vi "WaveSynthV2.vi"(6 "error in":errorcluster, 9 "Default Wave":bool) -> (0 "error out":errorcluster, 1 "Waves per Pixel 2":u32, 2 "Sampling Frequency (Hz) 2":u64, 3 "Amplitudes":dbl[](array[numeric]) format="%.2f", 4 "Offset Factor 2":dbl, 5 "Gain":dbl)   [LabVIEW 2020]
uses:
  WaveFormsAvailable.ctl
  <vilib>/Utility/file.llb/Read Delimited Spreadsheet (DBL).vi
  <vilib>/Utility/file.llb/Write Delimited Spreadsheet (DBL).vi
  <vilib>/Analysis/NI_AALBase.lvlib
panel:
  in  "Developers Option Control":enum32{"Dev"}(tab)
  out "Time Series":dbl[](array[numeric])
  in  "Wave View":enum32{"Single", "Complete Wave"}(tab)
  out "Single Wave":cluster{"tv":dbl[], dbl[]}(graph)
  out "Wave per Pixel":cluster{dbl[], dbl[]}(graph)
  in  "Save Button":bool
  in  "Start Time (us)":dbl=-0.2 format="%#_6p"
  in  "Number of Samples":u32=2048
  in  "Waveform Path":path
  in  "Sampling Frequency (Hz)":u64=200000000 format="%.2p"
  in  "Waves per Pixel":u32=1
  in  "Delay between waves (us)":dbl
  in  "Frequency (Hz)":u64=40000000 format="%.0p"
  in  "Wave":T1=enum."Ricker"
  in  "Reset Button":bool
  in  "Gain Factor":dbl=1.0
  in  "Offset Factor":dbl
  in  "Phase Delay (Samples)":i32
  in  "Done":bool
  # "Waveform Synthesizer"
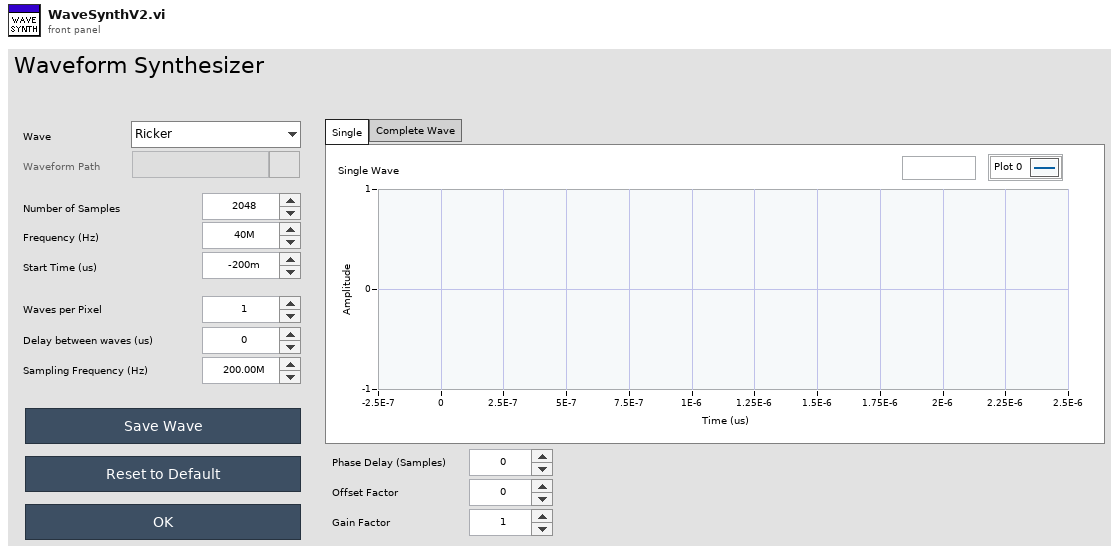
[diagram p1: front panel]
types:
  T1 = typedef "WaveFormsAvailable.ctl" = enum16{"Chirp", "Ricker", "Other..."}
  T2 = enum8{"Enabled", "Disabled", "Disabled and Grayed Out"}
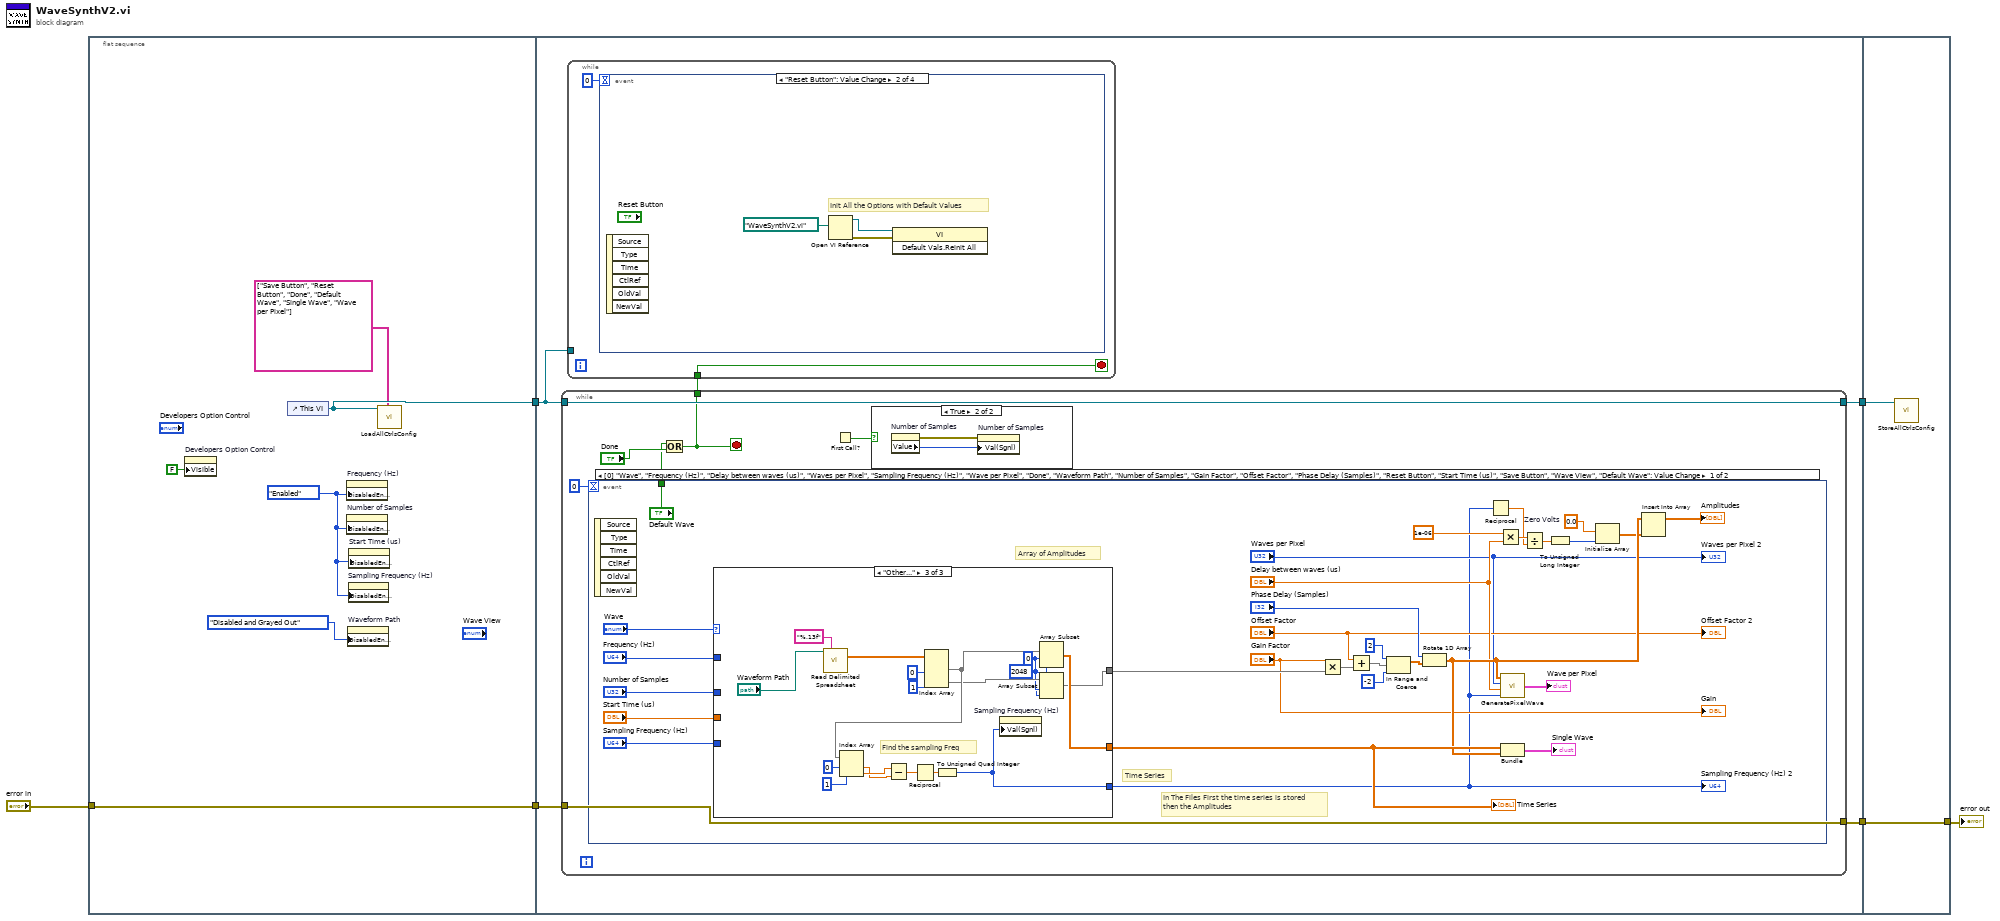
[diagram p0: block diagram]
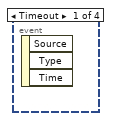
[diagram p2: hidden frame]
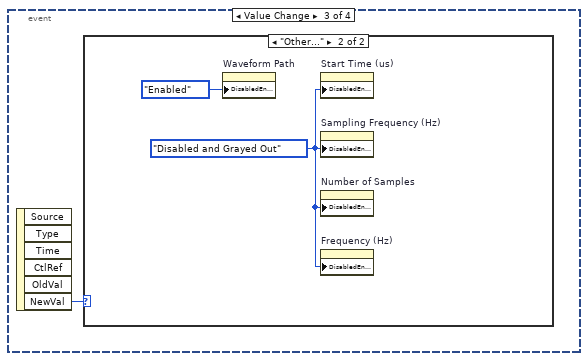
[diagram p3: hidden frame]
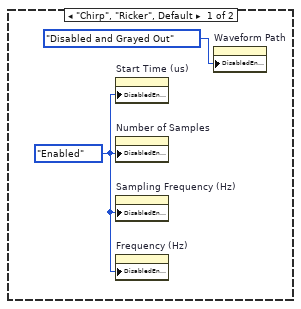
[diagram p4: hidden frame]
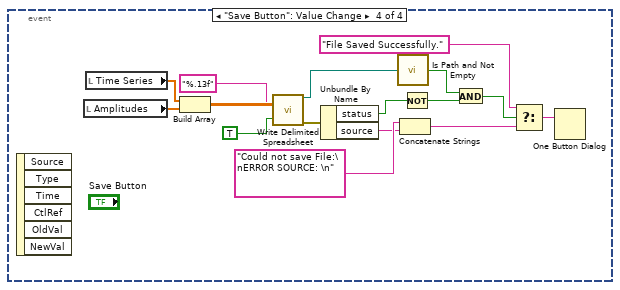
[diagram p5: hidden frame]
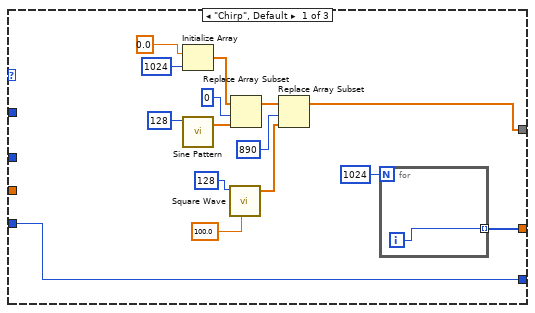
[diagram p7: hidden frame]
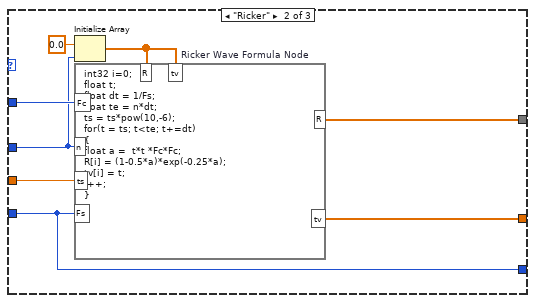
[diagram p8: hidden frame]
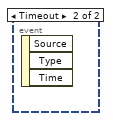
[diagram p9: hidden frame]
diagram:
  n1 = flat-sequence {
    tunnel: [w12] -> w3
    tunnel: [w11] -> w2
    tunnel: "error in" -> [w11]
    tunnel: [w17] -> w5
    tunnel: [w16] -> w4
    tunnel: w3 -> [w15]
    tunnel: w2 -> [w13]
    tunnel: [w126] -> w6
    tunnel: w5 -> [w126]
    tunnel: w4 -> [w125]
    frame #0 {
      w10 = T2."Enabled" ("Disabled")
      n2 = property on="Developers Option Control" class="TabCtl (strict)"("Visible"=FALSE) -> ()  [unwired: 2 in, 2 out]
      n3 = control-ref of="This VI"() -> (w12:refnum<vi>)
      n4 = property on="Frequency (Hz)" class="DigNum (strict)"("DisabledEnum"=w10) -> ()  [unwired: 2 in, 2 out]
      n5 = property on="Number of Samples" class="DigNum (strict)"("DisabledEnum"=w10) -> ()  [unwired: 2 in, 2 out]
      n6 = property on="Waveform Path" class="Path"("DisabledEnum"=T2."Disabled and Grayed Out" ("Disabled")) -> ()  [unwired: 2 in, 2 out]
      n7 = property on="Sampling Frequency (Hz)" class="DigNum (strict)"("DisabledEnum"=w10) -> ()  [unwired: 2 in, 2 out]
      n8 = property on="Start Time (us)" class="DigNum (strict)"("DisabledEnum"=w10) -> ()  [unwired: 2 in, 2 out]
      n9 = call "LoadAllCtrlsConfig.vi"("ExcludeLabels"=string[] ["Save Button", "Reset Button", "Done", "Default Wave", "Single Wave", "Wave per Pixel"], "VI in"=w12) -> ()  [unwired: 10 in]
    }
    frame #1 {
      n10 = while {
        tunnel: w13 -> [w50]
        tunnel: [w50] -> w17
        tunnel: w15 -> [w48]
        tunnel: [w48] -> w16
        tunnel: [w46] -> w14
        stop <- w46 stop-if-true
        n11 = event shown="[0] \"Wave\", \"Frequency (Hz)\", \"Delay between waves (us)\", \"Waves per Pixel\", \"Sampling Frequency (Hz)\", \"Wave per Pixel\", \"Done\", \"Waveform Path\", \"Number of Samples\", \"Gain Factor\", \"Offset Factor\", \"Phase Delay (Samples)\", \"Reset Button\", \"Start Time (us)\", \"Save Button\", \"Wave View\", \"Default Wave\": Value Change" {
          selector: _ -> [_ _]
          dyn-events: _ -> [_ _]
          timeout: 0 -> [_ _]
          tunnel: ["Default Wave" _] -> w44
          event "Frequency (Hz)", "Delay between waves (us)", "Waves per Pixel", "Sampling Frequency (Hz)", "Wave per Pixel", "Done", "Waveform Path", "Number of Samples", "Gain Factor", "Offset Factor", "Phase Delay (Samples)", "Reset Button", "Start Time (us)", "Save Button", "Wave View", "Default Wave": Value Change {
            w63 = 0.0  # Zero Volts
            # "Time Series"
            # "In The Files First the time series is stored \nthen the Amplitudes"
            # "Array of Amplitudes"
            n12 = event-data() -> ()  [unwired: 1 in, 6 out]
            n13 = case shown="\"Other...\"" "Wave" {
              tunnel: [w83 w105 w121] -> w82
              tunnel: "Frequency (Hz)" -> [_ w104 _]
              tunnel: "Start Time (us)" -> [_ w103 _]
              tunnel: "Number of Samples" -> [_ w101 _]
              tunnel: [w86 w100 w120] -> w77
              tunnel: "Sampling Frequency (Hz)" -> [w85 w99 _]
              tunnel: [w85 w99 w123] -> w53
              frame "Chirp", Default {
                n14 = Initialize Array(0.0 ("element"), 1024 ("dimension size")) -> (w91:dbl[])
                n15 = call <vilib>:"Sine Pattern.vi"("samples"=128) -> ("Sinusoidal Pattern"=w90:dbl[])  [unwired: 3 in, 1 out]
                n16 = call <vilib>:"Square Wave.vi"("samples"=128, "duty cycle (%)"=100.0) -> ("square wave"=w95:dbl[])  [unwired: 4 in, 2 out]
                n17 = Replace Array Subset(array=w91, new element=w90, index=0) -> (w96:dbl[])
                n18 = Replace Array Subset(array=w96, new element=w95, index=890) -> (w86:dbl[])
                n19 = for {
                  N: 1024 -> [_]
                  tunnel: [w98] -> w83 mode=indexing
                  i -> [w98]
                }
              }
              frame "Ricker" {
                n20 = Initialize Array(0.0 ("element"), w101) -> (w102:dbl[])
                n21 = formula code="int32 i=0;\nfloat t;\nfloat dt = 1/Fs;\nfloat te = n*dt;\nts = ts*pow(10,-6);\nfor(t = ts; t<te; t+=dt)\n{ \nfloat a =  t*t *Fc*Fc;\nR[i] = (1-0.5*a)*exp(-0.25*a);\ntv[i] = t;\ni++;\n}" "Ricker Wave Formula Node"("Fc"=w104, "R"=w102, "ts"=w103, "n"=w101, "Fs"=w99, "tv"=w102) -> ("R"=w100:dbl[], "tv"=w105:dbl[])
              }
              frame "Other..." {
                w117 = 2048 ("length")
                w118 = 0 ("index")
                # "Find the sampling Freq"
                n22 = call-poly <vilib>:"Read Delimited Spreadsheet.vi"("file path (dialog if empty)"="Waveform Path", "format (%.3f)"="%.13f" ("format (%d)")) -> ("all rows"=w114:dbl[][])  [unwired: 8 in, 5 out]
                n23 = Index Array(array=w114, index (col) #1=0 ("index (row)"), index (col) #2=1 ("index (col)")) -> (element #1=w122:dbl[], element #2=w119:dbl[])  [unwired: 2 in]
                n24 = Index Array(array=w122, index #1=0 ("index"), index #2=1 ("index")) -> (element #1=w109:dbl, element #2=w110:dbl)
                n25 = Subtract(x=w110, y=w109) -> (x-y=w108:dbl)
                n26 = Reciprocal(x=w108) -> (1/x=w107:dbl)
                n27 = To Unsigned Quad Integer(1:w107) -> (0:w123:u64)
                n28 = property on="Sampling Frequency (Hz)" class="DigNum (strict)"("Val(Sgnl)"=w123) -> ()  [unwired: 2 in, 2 out]
                n29 = Array Subset(array=w122, index=w118, length=w117) -> (w121:dbl[])
                n30 = Array Subset(array=w119, index=w118, length=w117) -> (w120:dbl[])
              }
            }
            "Time Series" <- w82
            "Sampling Frequency (Hz) 2" <- w53
            n31 = Multiply(x="Gain Factor", y=w77) -> (x*y=w76:dbl[])
            n32 = Add(x="Offset Factor", y=w76) -> (x+y=w72:dbl[])
            n33 = In Range and Coerce(upper limit=2, x=w72, lower limit=-2) -> (coerced(x)=w73:dbl[])  [unwired: 1 out]
            n34 = Rotate 1D Array(1:w73, 2:"Phase Delay (Samples)") -> (0:w61:dbl[])
            n35 = Reciprocal(x=w53) -> (1/x=w62:dbl)
            n36 = Multiply(x=1e-06, y="Delay between waves (us)") -> (x*y=w65:dbl)
            n37 = Bundle("tv"=w82, w61) -> (→"Single Wave":cluster{"tv":dbl[], dbl[]})  [unwired: 1 in]
            n38 = call "GeneratePixelWave.vi"("Fs"=w53, "Delay between waves (us)"="Delay between waves (us)", "Waves per Pixel"="Waves per Pixel", "Single Wave"=w61) -> ("Pixel Wave"=→"Wave per Pixel":cluster{dbl[], "R":dbl[]})
            n39 = Divide(x=w65, y=w62) -> (x/y=w67:dbl)
            n40 = To Unsigned Long Integer(number=w67) -> (unsigned 32bit integer=w66:u32)
            n41 = Initialize Array(w63, w66) -> (w60:dbl[])
            n42 = Insert Into Array(array=w61, new element=w60) -> (→"Amplitudes":dbl[])  [unwired: 1 in]
            "Waves per Pixel 2" <- "Waves per Pixel"
            "Gain" <- "Gain Factor"
            "Offset Factor 2" <- "Offset Factor"
          }
          event Timeout {
            n43 = event-data() -> ()  [unwired: 1 in, 3 out]
          }
        }
        n44 = Or(x=w44, y="Done") -> (x .or. y?=w46:bool)
        n45 = First Call?() -> (First Call?: T/F=w45:bool)
        n46 = case shown="True" w45 {
          frame False {
          }
          frame True {
            n47 = property on="Number of Samples" class="DigNum (strict)"() -> (error out=w51:errorcluster, "Value"=w52:u32)  [unwired: 2 in, 1 out]
            n48 = property on="Number of Samples" class="DigNum (strict)"(error in=w51, "Val(Sgnl)"=w52) -> ()  [unwired: 1 in, 2 out]
          }
        }
      }
      n49 = while {
        tunnel: w15 -> [_]
        tunnel: w14 -> [w18]
        stop <- w18 stop-if-true
        n50 = event shown="[1] \"Reset Button\": Value Change" {
          selector: _ -> [_ _ _ _]
          dyn-events: _ -> [_ _ _ _]
          timeout: 0 -> [_ _ _ _]
          event Timeout {
            n51 = event-data() -> ()  [unwired: 1 in, 3 out]
          }
          event "Reset Button": Value Change {
            # "Init All the Options with Default Values"
            n52 = event-data() -> ()  [unwired: 1 in, 6 out]
            n53 = Open VI Reference(vi path=path "WaveSynthV2.vi") -> (vi reference=w21:refnum<vi>, error out=w22:errorcluster)  [unwired: 5 in]
            n54 = invoke class="VI" method="Default Vals.Reinit All"(reference=w21, error in=w22) -> ()  [unwired: 1 in, 3 out]
          }
          event Value Change {
            n55 = event-data() -> ("NewVal"=w23:T1)  [unwired: 1 in, 5 out]
            n56 = case shown="\"Other...\"" w23 {
              frame "Chirp", "Ricker", Default {
                w25 = T2."Enabled" ("Disabled")
                n57 = property on="Start Time (us)" class="DigNum (strict)"("DisabledEnum"=w25) -> ()  [unwired: 2 in, 2 out]
                n58 = property on="Number of Samples" class="DigNum (strict)"("DisabledEnum"=w25) -> ()  [unwired: 2 in, 2 out]
                n59 = property on="Sampling Frequency (Hz)" class="DigNum (strict)"("DisabledEnum"=w25) -> ()  [unwired: 2 in, 2 out]
                n60 = property on="Frequency (Hz)" class="DigNum (strict)"("DisabledEnum"=w25) -> ()  [unwired: 2 in, 2 out]
                n61 = property on="Waveform Path" class="Path"("DisabledEnum"=T2."Disabled and Grayed Out" ("Disabled")) -> ()  [unwired: 2 in, 2 out]
              }
              frame "Other..." {
                w27 = T2."Disabled and Grayed Out" ("Disabled")
                n62 = property on="Waveform Path" class="Path"("DisabledEnum"=T2."Enabled" ("Disabled")) -> ()  [unwired: 2 in, 2 out]
                n63 = property on="Start Time (us)" class="DigNum (strict)"("DisabledEnum"=w27) -> ()  [unwired: 2 in, 2 out]
                n64 = property on="Sampling Frequency (Hz)" class="DigNum (strict)"("DisabledEnum"=w27) -> ()  [unwired: 2 in, 2 out]
                n65 = property on="Number of Samples" class="DigNum (strict)"("DisabledEnum"=w27) -> ()  [unwired: 2 in, 2 out]
                n66 = property on="Frequency (Hz)" class="DigNum (strict)"("DisabledEnum"=w27) -> ()  [unwired: 2 in, 2 out]
              }
            }
          }
          event "Save Button": Value Change {
            n67 = event-data() -> ()  [unwired: 1 in, 6 out]
            n68 = local read "Amplitudes"() -> (w29:dbl[])
            n69 = local read "Time Series"() -> (w30:dbl[])
            n70 = Build Array(w30, w29) -> (w43:dbl[][])
            n71 = call-poly <vilib>:"Write Delimited Spreadsheet.vi"("format (%.3f)"="%.13f", "2D data"=w43, "transpose? (no:F)"=TRUE) -> ("new file path (Not A Path if cancelled)"=w35:path, "error out"=w39:errorcluster)  [unwired: 11 in]
            n72 = Unbundle By Name(w39) -> ("status"=w34:bool, "source"=w36:string)
            n73 = call <vilib>:"Is Path and Not Empty.vi"("path"=w35) -> ("Is Path and Not Empty?"=w33:bool)  [unwired: 4 in]
            n74 = Concatenate Strings("Could not save File:\nERROR SOURCE: \n", w36) -> (w37:string)
            n75 = Not(x=w34) -> (.not. x?=w31:bool)
            n76 = And(x=w33, y=w31) -> (x .and. y?=w32:bool)
            n77 = Select(t="File Saved Successfully.", s=w32, f=w37) -> (s? t:f=w41:string)
            n78 = One Button Dialog(message=w41) -> ()  [unwired: 1 in, 1 out]
          }
        }
      }
    }
    frame #2 {
      n79 = call "StoreAllCtrlsConfig.vi"("VI in"=w125) -> ()  [unwired: 11 in]
    }
  }
  "error out" <- w6
